vi "Write Drive Train Status.vi"(8 "error in (no error)":errorcluster, 10 "Drive Train Status":T1 {"Right Power Setpoint" min=-1.0 max=1.0 step=0.1 scale=-1.0..1.0; "Left Power Setpoint" min=-1.0 max=1.0 step=0.1 scale=-1.0..1.0; "Right Power" min=-1.0 max=1.0 step=0.1 scale=-1.0..1.0; "Left Power" min=-1.0 max=1.0 step=0.1 scale=-1.0..1.0}, 11 "Drive Train in":refnum<class "Drive Train.lvclass">) -> (0 "error out":errorcluster, 3 "Drive Train out":refnum<class "Drive Train.lvclass">)   [LabVIEW 2014, in "Logical Systems.lvlib" / "Drive Train.lvlib" / "Drive Train.lvclass"]
uses:
  Drive Train.lvclass
  Drive Train Status.ctl
  Drive Train.lvclass/Drive Train.ctl
  Drive Train Commands/Drive Train Command/Drive Train Command Messages/New Drive Train Status Msg/New Drive Train Status Msg.lvclass/New Drive Train Status Msg.ctl
  <vilib>/ActorFramework/Message Enqueuer/Message Enqueuer.lvclass/Message Enqueuer.ctl
  <vilib>/ActorFramework/Message Enqueuer/Enqueue.vi
  <vilib>/ActorFramework/Message Priority Queue/Priority Enqueue.vi
  Drive Train Commands/Drive Train Command/Drive Train Command Messages/New Drive Train Status Msg/New Drive Train Status Msg.lvclass
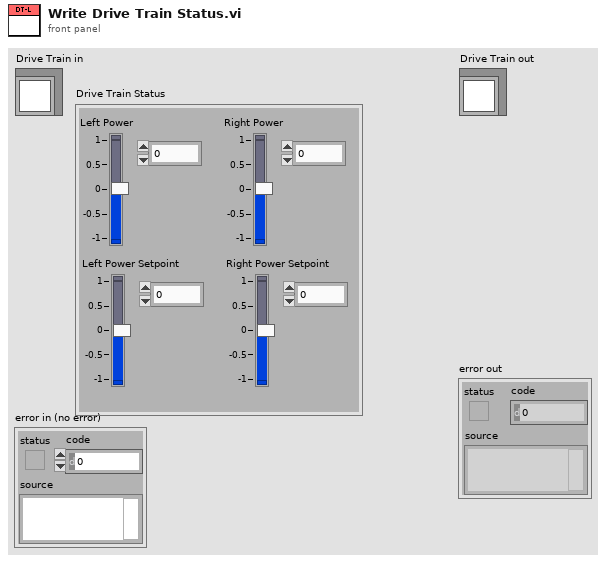
[diagram p1: front panel]
types:
  T1 = typedef "Logical Systems.lvlib/Drive Train.lvlib/Drive Train.lvclass/Drive Train Status.ctl" = cluster{"Left Power":dbl, "Right Power":dbl, "Left Power Setpoint":dbl, "Right Power Setpoint":dbl}
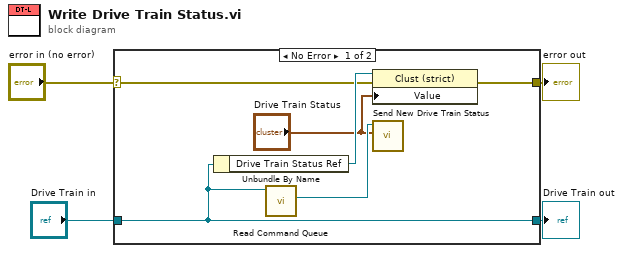
[diagram p0: block diagram]
diagram:
  n1 = case shown="No Error" "error in (no error)" {
    selector: "error in (no error)" -> [w9 w12]
    tunnel: [w8 w12] -> w3
    tunnel: [w7 w11] -> w1
    tunnel: "Drive Train in" -> [w7 w11]
    frame No Error {
      n2 = Unbundle By Name(w7) -> ("Drive Train Status Ref"=w10:refnum<vi>)
      n3 = call-dynamic "Read Command Queue.vi"("System Actor in"=w7) -> ("Actor Framework:Message Enqueuer"=w6:refnum<class "Message Enqueuer.lvclass">)  [unwired: 8 in, 2 out]
      n4 = property class="Clust (strict)"(reference=w10, error in=w9, "Value"="Drive Train Status") -> (error out=w8:errorcluster)  [unwired: 1 out]
      n5 = call "Send New Drive Train Status.vi"("Drive Train Status"="Drive Train Status", "Message Enqueuer"=w6) -> ()  [unwired: 8 in, 2 out]
    }
    frame Error {
    }
  }
  "error out" <- w3
  "Drive Train out" <- w1
